vi "Band Phase (Frequency).vi"(0 "Cross phase [degrees]":cluster{"f0":dbl, "df":dbl, "phase":sgl[]}, 5 "Start":dbl, 7 "Stop":dbl, 11 "error in (no error)":errorcluster) -> (6 "Phase (deg)":sgl, 15 "error out":errorcluster)   [LabVIEW 2017, in "VibrationAnalysisFunctions.lvlib"]
uses:
  <vilib>/addons/InsightCM/Utilities/Analysis/Vibration/VibrationAnalysisFunctions.lvlib
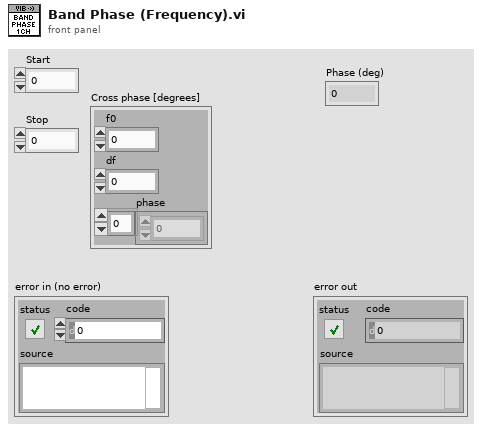
[diagram p1: front panel]
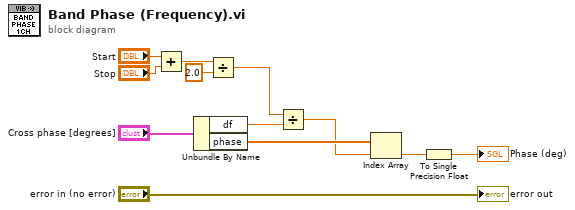
[diagram p0: block diagram]
diagram:
  n1 = Add(x="Start", y="Stop") -> (x+y=w5:dbl)
  n2 = Unbundle By Name("Cross phase [degrees]") -> ("df"=w2:dbl, "phase"=w9:sgl[])
  n3 = Divide(x=w5, y=2.0) -> (x/y=w3:dbl)
  n4 = Divide(x=w3, y=w2) -> (x/y=w1:dbl)
  n5 = Index Array(array=w9, index=w1) -> (element=w8:sgl)
  n6 = To Single Precision Float(number=w8) -> (single precision float=→"Phase (deg)":sgl)
  "error out" <- "error in (no error)"
